vi "LNLS Control BPM Data.vi"(8 "error in (no error)":errorcluster, 10 "BPM Status (On correction?)":bool[](array[boolean]), 11 "BPM Readings":dbl[](array[numeric])) -> (0 "error out":errorcluster, 3 "BPM Readings Data":T1[](array[typedef]) {"status" format="%08b"})   [LabVIEW 2011, in "LNLS Control VIs.lvlib"]
uses:
  LNLS Control VIs.lvlib
  Types Definitions/Type BPM Pre Encode.ctl
  Type Definitions.lvlib
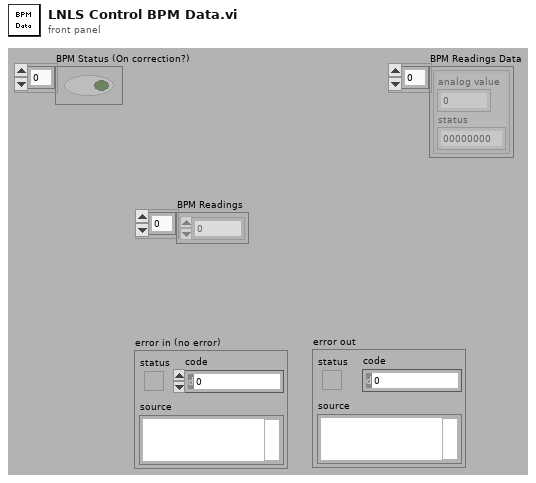
[diagram p1: front panel]
types:
  T1 = typedef "Type Definitions.lvlib/Type BPM Pre Encode.ctl" = cluster{"analog value":dbl, "status":u8}
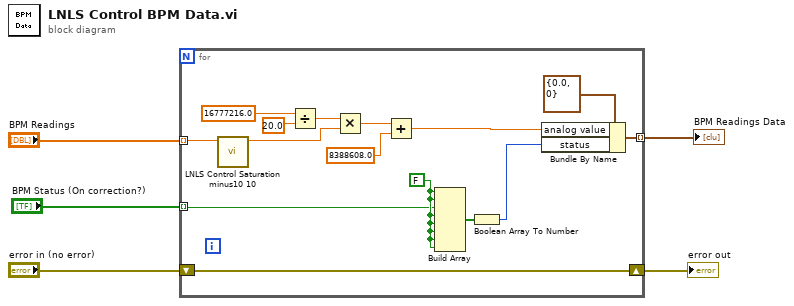
[diagram p0: block diagram]
diagram:
  n1 = for {
    tunnel: [w20] -> w2 mode=indexing
    shift-right: [w19] -> w4
    shift-left: "error in (no error)" -> [w19]
    tunnel: "BPM Readings" -> [w8] mode=indexing
    tunnel: "BPM Status (On correction?)" -> [w10] mode=indexing
    w11 = FALSE ("element")
    n2 = call "LNLS Control Saturation minus10 10.vi"("in"=w8) -> ("saturated out"=w7:dbl)  [unwired: 10 in]
    n3 = Divide(x=16777216.0, y=20.0) -> (x/y=w13:dbl)
    n4 = Multiply(x=w13, y=w7) -> (x*y=w15:dbl)
    n5 = Add(x=w15, y=8388608.0) -> (x+y=w6:dbl)
    n6 = Build Array(w11, w11, w10, w11, w11, w11, w11, w11) -> (w12:bool[])
    n7 = Boolean Array To Number(Boolean array=w12) -> (number=w9:u32)
    n8 = Bundle By Name(cluster=T1 {"analog value"=0.0, "status"=0} ("LOCON_BIPOLAR_16BITS"), "analog value"=w6, "status"=w9) -> (w20:T1)
  }
  "error out" <- w4
  "BPM Readings Data" <- w2
